vi "WaitForAsyncReturnData.vi"(8 "error in (no error)":errorcluster, 10 "timeout in ms (-1)":i32=-1, 11 "SMO":refnum<class "SMO.lvclass">) -> (0 "error out":errorcluster, 2 "Process Notification":T1, 3 "SMO out":refnum<class "SMO.lvclass">)   [LabVIEW 2019, in "SMO.lvclass"]
doc: "JKI State Machine Objects (SMO) 1.3.0.56\nJKI - JKI\nCopyright (c) 2017, JKI"
uses:
  SMO.lvclass
  Typedefs/Process Error Notification--Cluster.ctl
  SMO.lvclass/SMO.ctl
panel:
  # "For instructions on how to use the JKI State Machine Objects, examples and video tutorials, visit:\nhttp://jki.net/state-machine-objects/\n\nJKI State Machine Objects™\nhttp://jki.net/state-machine-objects/\nCopyright (C) 2005-2015, JKI <info@jki.net>\nALL RIGHTS RESERVED"
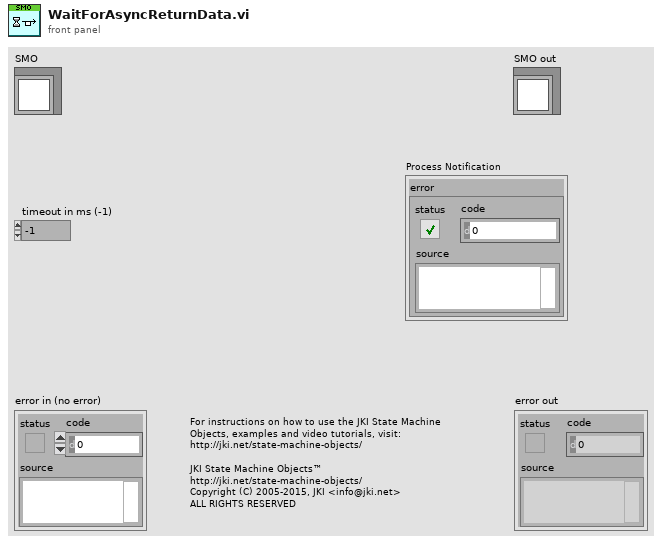
[diagram p1: front panel]
types:
  T1 = typedef "SMO.lvclass/Process Error Notification--Cluster.ctl" = cluster{"error":errorcluster}
  T2 = typedef "SMO.lvclass/PrivateData--Ref.ctl" = refnum<data-value>
  T3 = typedef "SMO.lvclass/PrivateData--Cluster.ctl" = cluster{"Parent Call":T4, "Registered Processes":T5[], "Sync Notifier":refnum<notifier>, "Process Error Notifier":refnum<notifier>, "Protected Events":T6, "Public Events":T7, "SMO State":T8, "[Dependencies]":T9[], "[Attributes]":refnum<class "Attribute.lvclass">[], "Launcher Close":refnum<notifier>, "Caller Watchdog":refnum<queue>, "Accessibility":T10, "NbStaticDependencies":u32}
  T4 = typedef "SMO.lvclass/Parent Call--Enum.ctl" = enum16{"Allows parent to run", "Does not request parent to run"}
  T5 = typedef "SMO.lvclass/RegisteredProcessData--Cluster.ctl" = cluster{"Name":string, "Static VI Ref":refnum<vi>, "Running":bool, "NotifierRef":u32}
  T6 = typedef "SMO.lvclass/Protected Events.ctl" = cluster{"StopProcesses":refnum<user-event>, "AbortProcesses":refnum<user-event>, "Config Changed":refnum<user-event>, "Dependency":refnum<user-event>}
  T7 = typedef "SMO.lvclass/Public Events.ctl" = cluster{"Error":refnum<user-event>, "State":refnum<user-event>, "Reserve State":refnum<user-event>}
  T8 = typedef "SMO.lvclass/SMOState --Enum.ctl" = enum16{"unknown", "Created", "Started", "Stopped"}
  T9 = typedef "SMO.lvclass/SMO Dependency--Cluster.ctl" = cluster{"Dependency":refnum<class "SMO.lvclass">, "Level":string}
  T10 = typedef "SMO.lvclass/Accessibility--Cluster.ctl" = cluster{"Lock Key":string, "Reserve State":T11}
  T11 = typedef "SMO.lvclass/Reserve State--Enum.ctl" = enum16{"Unreserved", "Reserved", "Self-locked"}
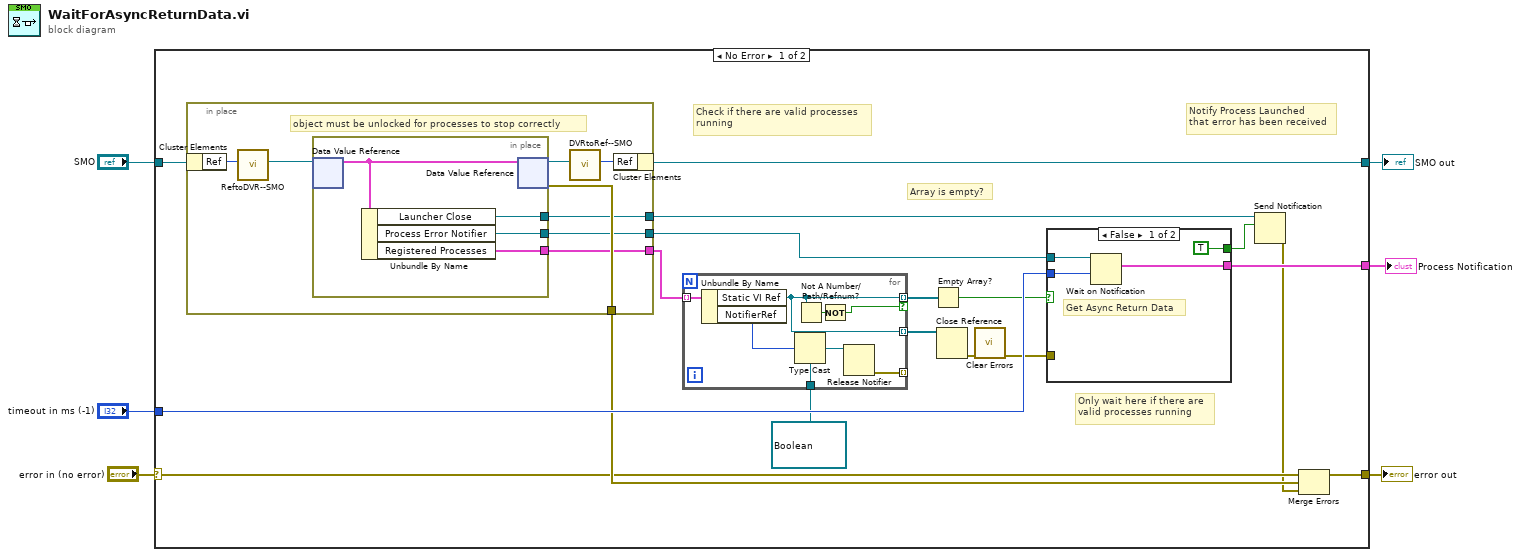
[diagram p0: block diagram]
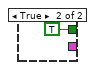
[diagram p2: hidden frame]
diagram:
  n1 = case shown="No Error" "error in (no error)" {
    selector: "error in (no error)" -> [w19 w51]
    tunnel: "timeout in ms (-1)" -> [w23 _]
    tunnel: [w21 w51] -> w5
    tunnel: "SMO" -> [w20 w50]
    tunnel: [w16 w50] -> w2
    tunnel: [w15 _] -> w1
    frame No Error {
      # "Notify Process Launched\nthat error has been received"
      # "Check if there are valid processes\nrunning"
      # "Array is empty?"
      # "Only wait here if there are\nvalid processes running"
      n2 = in-place {
        in-place-border: [w45] -> w22
        in-place-border: [w44] -> w24
        in-place-border: [w43] -> w18
        in-place-border: [w38] -> w14
        # "object must be unlocked for processes to stop correctly"
        n3 = in-place-cluster #1(w20) -> ("Ref"=w42:u32)
        n4 = call "ReftoDVR--SMO.vi"("Ref"=w42) -> ("Ref"=w41:T2)  [unwired: 10 in]
        n5 = in-place {
          in-place-border: [w48] -> w44
          in-place-border: [w47] -> w43
          in-place-border: [w46] -> w38
          n6 = in-place-dvr #2(w41) -> (w49:T3)  [unwired: 1 out]
          n7 = Unbundle By Name(w49) -> ("Launcher Close"=w46:refnum<notifier>, "Process Error Notifier"=w48:refnum<notifier>, "Registered Processes"=w47:T5[])
          n8 = in-place-dvr #2(w49) -> (w40:T2, w45:errorcluster)
        }
        n9 = call "DVRtoRef--SMO.vi"("Ref"=w40) -> ("Ref"=w39:u32)  [unwired: 10 in]
        n10 = in-place-cluster #1("Ref"=w39) -> (w16:refnum<class "SMO.lvclass">)
      }
      n11 = for {
        tunnel: w18 -> [w30] mode=indexing
        tunnel: [w29] -> w11 mode=indexing if=w31
        tunnel: [w29] -> w8 mode=indexing
        tunnel: refnum<notifier> refnum ("notifier") -> [w27]
        tunnel: [w25] -> _ mode=indexing
        n12 = Unbundle By Name(w30) -> ("Static VI Ref"=w29:refnum<vi>, "NotifierRef"=w28:u32)
        n13 = Type Cast(type=w27, x=w28) -> (*(type *) &x=w26:refnum<notifier>)
        n14 = Not A Number/Path/Refnum?(number/path/refnum=w29) -> (NaN/Path/Refnum?=w32:bool)
        n15 = Not(x=w32) -> (.not. x?=w31:bool)
        n16 = Release Notifier(notifier=w26) -> (error out=w25:errorcluster)  [unwired: 2 in, 2 out]
      }
      n17 = Empty Array?(array=w11) -> (empty?=w17:bool)
      n18 = Close Reference(reference=w8) -> (error out=w9:errorcluster)  [unwired: 1 in]
      n19 = call <vilib>:"Clear Errors.vi"("error in (no error)"=w9) -> ("error out"=w10:errorcluster)  [unwired: 5 in, 1 out]
      n20 = case shown="False" w17 {
        tunnel: w23 -> [w36 _]
        tunnel: [w34 _] -> w15
        tunnel: w24 -> [w35 _]
        tunnel: [TRUE ("ignore previous (F)") TRUE ("ignore previous (F)")] -> w13
        tunnel: w10 -> [_ _]
        frame False {
          # "Get Async Return Data"
          n21 = Wait on Notification(notifier=w35, timeout in ms (-1)=w36) -> (notification=w34:T1)  [unwired: 2 in, 3 out]
        }
        frame True {
        }
      }
      n22 = Send Notification(notification=w13, notifier=w14) -> (error out=w12:errorcluster)  [unwired: 1 in, 1 out]
      n23 = Merge Errors(w19, w22, w12) -> (w21:errorcluster)
    }
    frame Error {
    }
  }
  "SMO out" <- w2
  "error out" <- w5
  "Process Notification" <- w1
